vi "AlliGator Run XY Graph Python Function (API v1).vi"(6 "Mouse Click Event Data":T1, 7 "AlliGator Ctrl Refnums":T8, 8 "error in (no error)":errorcluster, 9 "data value reference in":refnum<data-value>, 10 "Python Function Info":T4, 11 "Python Session ID":refnum<k35>) -> (0 "error out":errorcluster, 1 "Data Value Reference out":refnum<data-value>, 2 "JSON String":string, 3 "Function Display Name":string, 4 "Function Parameters JSON String":string, 5 "Message":string)   [LabVIEW 2021, in "AlliGator Python Plugins.lvlib"]
uses:
  AlliGator Python Plugins.lvlib
  GUI/AlliGator Ctrl Refnums.ctl
  GUI/AlliGator Other Ctrl Refnums.ctl
  GUI/AlliGator State Indicator.ctl
  GUI/AlliGator Main Window Tabs.ctl
  GUI/AlliGator Phasor Plot Ctrl Refnums.ctl
  GUI/AlliGator Phasor Graph Ctrl Refnums.ctl
  Phasor/Phasor Calibration Type.ctl
  GUI/AlliGator Dataset Ctrl Refnums.ctl
  Source Image/AlliGator Displayed Image.ctl
  GUI/AlliGator Registered Events Ctrl Refnums.ctl
  GUI/AlliGator Image Histogram Control Refnums.ctl
  Histograms/Linear Histogram Options.ctl
  Histograms/Histogram Bin Option.ctl
  Histograms/Histogram Bin Position.ctl
  Decay Fit Parameter Map/AlliGator Decay Fit Map Control Refnums.ctl
  Fits/IRF(X)PSED/Decay Fit Parameters & Derived Quantities List v2.ctl
  Parameter Map/AlliGator Parameter Map Control Refnums.ctl
  Internal Variables/AlliGator Internal Variables v2.ctl
  <vilib>/vision/Image Controls.llb/IMAQ Image.ctl
  Internal Variables/AlliGator Gate Image Set.ctl
  Files/AlliGator FLI Dataset Type.ctl
  Files/AlliGator Data Series Type.ctl
  Dual-Channel Datasets/AlliGator Dataset Channel.ctl
  Settings/AlliGator Gate Arithmetic.ctl
  Image/Named ROI Description.ctl
  Phasor Graph/AlliGator Decay Metadata v3.ctl
  Decay Analysis/Decay Preprocessing/AlliGator Decay Background Subtraction Info.ctl
  Decay Analysis/Decay Preprocessing/AlliGator Baseline Subtraction Method.ctl
  Graphs/XY Graph/XY Graph Plot Shift Parameters.ctl
  Graphs/XY Graph/XY Graph Plot Shift Method.ctl
  Decay Analysis/Decay Preprocessing/AlliGator Decay Extrapolation Parameters.ctl
  Phasor/Calibration Phasor (m, phi).ctl
  Phasor/Phasor Reference Series.ctl
  Phasor/Phasor Calibration Map v2.ctl
  Phasor/Phasor (g, s).ctl
  Phasor Graph/AlliGator Raw Phasor Plot Data v5.ctl
  Phasor/Phasor Standard Deviation Options.ctl
  Phasor Plot/AlliGator Phasor Multi-Harmonic Data.ctl
  Phasor/Phasor Harmonic Data.ctl
  Decay Fit Parameter Map/AlliGator Decay Fit Options & Parameters v4.ctl
  Fits/IRF(X)PSED/Decay Fit Options v4.ctl
  Fits/Decay Convolution/Decay Model.ctl
  Fits/Residual Type.ctl
  Fits/IRF(X)PSED/Fit Weights Type v2.ctl
  Fits/Non-linear Fitting Method v2.ctl
  Fits/Fit Calculation Method.ctl
  Fits/Non-linear Fitting Algorithm.ctl
  Decay Analysis/Decay Fit/AlliGator Decay Fit Parameter Constraints 2.ctl
  Fits/IRF(X)PSED/Decay Fit Parameters In List.ctl
  Fits/IRF(X)PSED/MLE Baseline Offset Type.ctl
  Decay Analysis/Decay Preprocessing/AlliGator Decay Preprocessing Parameters.ctl
  Fits/IRF(X)PSED/Decay Fit Result Constraint.ctl
  Decay Fit Parameter Map/AlliGator Parameter Maps Data.ctl
  AlliGator Python Function Information.ctl
  AlliGator Python Function Parameter Definition.ctl
  AlliGator Python Function Output Definition.ctl
  AlliGator Python Plugin Target Type.ctl
  Graphs/XY Graph/XY Graph Mouse Click Event Data.ctl
  Graphs/XY Graph/XY Graph Refnum.ctl
  <vilib>/Utility/miscctls.llb/LVPoint32TypeDef.ctl
  AlliGator Python Plugin Plot Data v1.ctl
  AlliGator Python Plugin Graph Data v1.ctl
  Graphs/Get Plot at Mouse Click (XY Graph)/Get Plot at Mouse Click [AAC].vi
  Graphs/Graphs.lvlib
  Graphs/XY Graph/XY Graph Add-Ons.lvlib
  Strings/Strings.lvlib
  GUI/AlliGator GUI.lvlib
  Error/Error.lvlib
  Source Image/AlliGator Source Image.lvlib
  Phasor/Phasor.lvlib
  Histograms/Histogram Window.lvlib
  Fits/Fits.lvlib
  Decay Fit Parameter Map/AlliGator Decay Fit Parameter Map.lvlib
  Parameter Map/AlliGator Parameter Map.lvlib
  Image/Image.lvlib
  Decay Analysis/Decay Preprocessing/AlliGator Decay Preprocessing.lvlib
  Phasor Graph/AlliGator Phasor Graph.lvlib
  Files/AlliGator Files.lvlib
  Internal Variables/AlliGator Internal Variables.lvlib
  Phasor Plot/AlliGator Phasor Plot.lvlib
  Decay Analysis/Decay Fit/AlliGator Decay Fit.lvlib
  Settings/AlliGator Settings.lvlib
  Dual-Channel Datasets/AlliGator Dual-Channel Datasets.lvlib
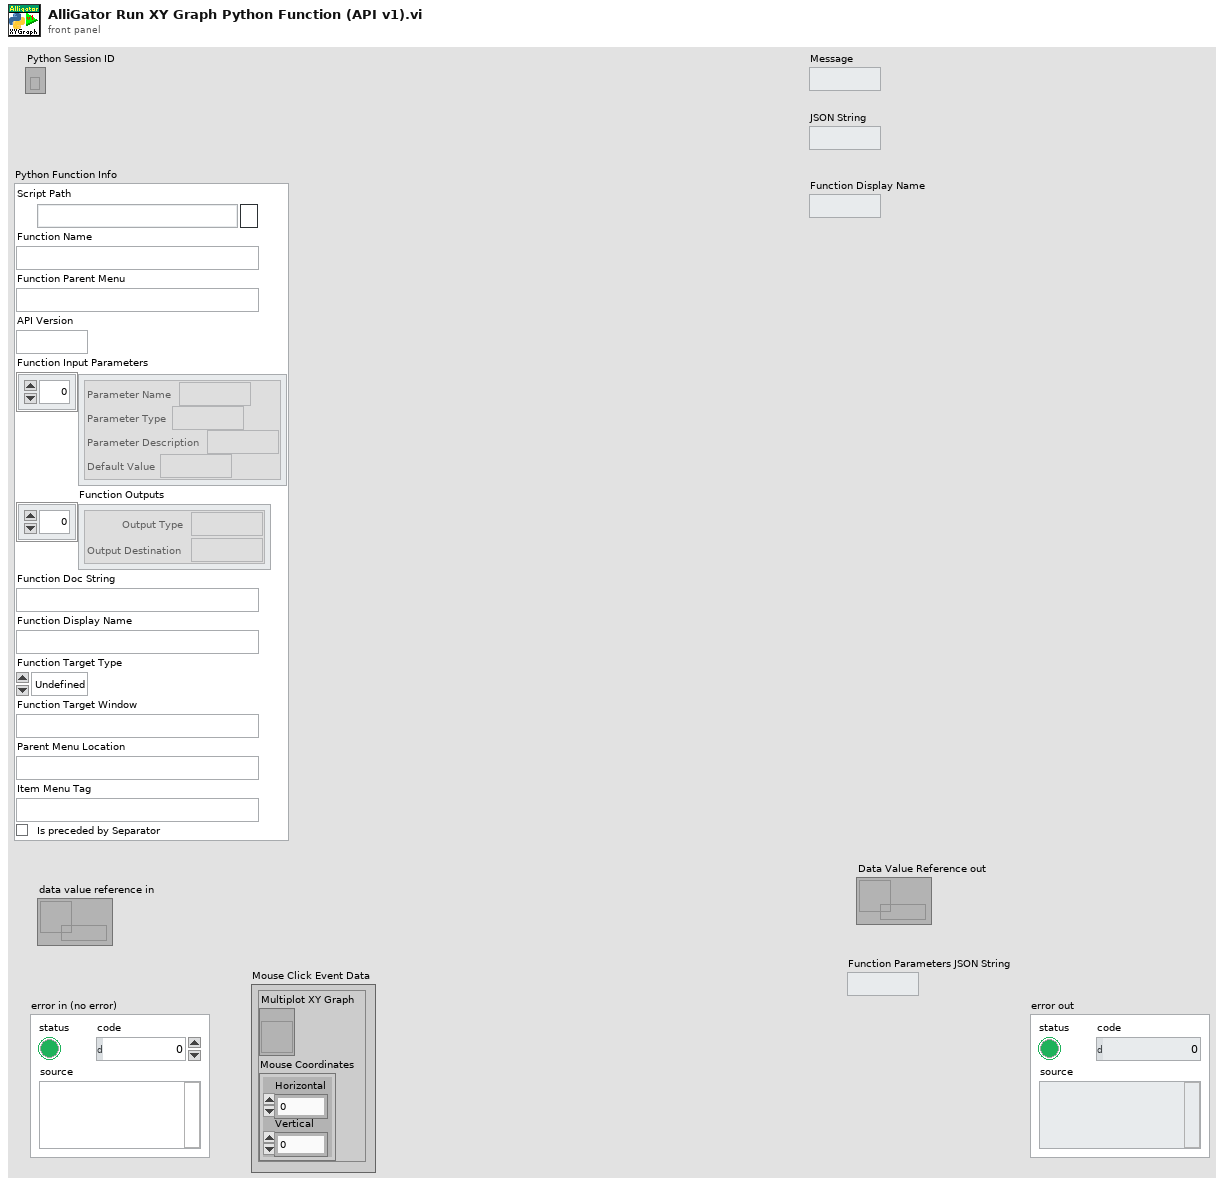
[diagram p1: front panel]
types:
  T1 = typedef "XY Graph Add-Ons.lvlib/XY Graph Mouse Click Event Data.ctl" = cluster{"Multiplot XY Graph":T2, "Mouse Coordinates":T3}
  T2 = typedef "XY Graph Add-Ons.lvlib/XY Graph Refnum.ctl" = refnum<vi>
  T3 = typedef "LVPoint32TypeDef.ctl" = cluster{"Horizontal":i32, "Vertical":i32}
  T4 = typedef "AlliGator Python Plugins.lvlib/AlliGator Python Function Information.ctl" = cluster{"Script Path":path, "Function Name":string, "Function Parent Menu":string, "API Version":string, "Function Input Parameters":T5[], "Function Outputs":T6[], "Function Doc String":string, "Function Display Name":string, "Function Target Type":T7, "Function Target Window":string, "Parent Menu Location":string, "Item Menu Tag":string, "Is preceded by Separator":bool}
  T5 = typedef "AlliGator Python Plugins.lvlib/AlliGator Python Function Parameter Definition.ctl" = cluster{"Parameter Name":string, "Parameter Type":string, "Parameter Description":string, "Default Value":string}
  T6 = typedef "AlliGator Python Plugins.lvlib/AlliGator Python Function Output Definition.ctl" = cluster{"Output Type":string, "Output Destination":string}
  T7 = typedef "AlliGator Python Plugins.lvlib/AlliGator Python Plugin Target Type.ctl" = enum16{"Undefined", "Window Menu", "Object Menu"}
  T8 = typedef "AlliGator GUI.lvlib/AlliGator Ctrl Refnums.ctl" = cluster{"Other AlliGator Ctrl Refnums":T9, "Phasor Plot Ctrl Refnums":T10, "Phasor Graph Ctrl Refnums":T11, "Dataset Control Refnums":T12, "Registered Events Ctrl Refnums":T13, "Image Histogram Ctrl Refnums":T14, "Decay Fit Map Ctrl Refnums":T15, "Parameter Map Ctrl Refnums":T16}
  T9 = typedef "AlliGator GUI.lvlib/AlliGator Other Ctrl Refnums.ctl" = cluster{"State Indicators":refnum<vi>, " Progress Bar":refnum<vi>, "Decay Graph Active":refnum<vi>, "Decay Statistics Bin":refnum<vi>, "Time Step":refnum<vi>, "Use File Timestamp":refnum<vi>, "Tab Control":refnum<vi>, "CPU":refnum<vi>, "Abort Fit":refnum<vi>, "Dataset File/Folder Path":refnum<vi>, "Abort ROI Creation":refnum<vi>, "Event LED":refnum<vi>, "Dataset File/Folder Path 2":refnum<vi>, "Dataset File/Folder Path 3":refnum<vi>, "Dataset File/Folder Path 4":refnum<vi>, "Dataset File/Folder Path 5":refnum<vi>, "Dataset File/Folder Path 6":refnum<vi>, "Dataset File/Folder Path 7":refnum<vi>, "Dataset File/Folder Path 8":refnum<vi>, "Dataset File/Folder Path 9":refnum<vi>, "Dataset File/Folder Path 10":refnum<vi>, "Dataset File/Folder Path 11":refnum<vi>}
  T10 = typedef "AlliGator GUI.lvlib/AlliGator Phasor Plot Ctrl Refnums.ctl" = cluster{"Phasor Ratio":refnum<vi>, "Modulus Lifetime":refnum<vi>, "Phasor at cursor (m, phi)":refnum<vi>, "Phase Lifetime":refnum<vi>, "Phasor at cursor (g, s)":refnum<vi>, "Phasor Plor Average Lifetime":refnum<vi>, "Phasor Plot Active":refnum<vi>, "Save Phasor Plot":refnum<vi>, "Image Overlay Color":refnum<vi>, "Phasor Plot Color Scale":refnum<vi>, "Reference 1 Button":refnum<vi>, "Reference 2 Button":refnum<vi>, "True Phasor Plot Value":refnum<vi>}
  T11 = typedef "AlliGator GUI.lvlib/AlliGator Phasor Graph Ctrl Refnums.ctl" = cluster{"Phasor Ratio":refnum<vi>, "Modulus Lifetime":refnum<vi>, "Phasor at cursor (m, phi)":refnum<vi>, "Phase Lifetime":refnum<vi>, "Phasor at cursor (g, s)":refnum<vi>, "Phasor Graph Average Lifetime":refnum<vi>, "Phasor Graph Active":refnum<vi>, "Save Phasor Graph":refnum<vi>, "Phasor Frame Slide":refnum<vi>, "Single Step Phasor":refnum<vi>, "Calibration Type":refnum<vi>, "Show Line":refnum<vi>, "Phase Lifetime 1":refnum<vi>, "Phase Lifetime 2":refnum<vi>, "Phasor Graph Frequency":refnum<vi>, "Phasor Reference 1 Control":refnum<vi>, "Phasor Reference 2 Control":refnum<vi>, "Calibration Lifetime":refnum<vi>, "Phase Lifetime SDV":refnum<vi>, "Average Lifetime SDV":refnum<vi>, "Phasor Ratio SDV":refnum<vi>, "Modulus Lifetime SDV":refnum<vi>}
  T12 = typedef "AlliGator GUI.lvlib/AlliGator Dataset Ctrl Refnums.ctl" = cluster{"Current Data":refnum<vi>, "Gate Image Slide":refnum<vi>, "Time Point Slide":refnum<vi>, "Current Time Stamp":refnum<vi>, "Save Image":refnum<vi>, "Displayed Image":refnum<vi>, "Overlay Mode":refnum<vi>, "Phasor Overlay Color":refnum<vi>, "Image Color Scale":refnum<vi>, "Use ROI as Search Area":refnum<vi>, "Source Image ROI Color":refnum<vi>, "True Pixel Value":refnum<vi>}
  T13 = typedef "AlliGator GUI.lvlib/AlliGator Registered Events Ctrl Refnums.ctl" = cluster{"Time Point Slider":refnum<vi>, "Phasor Plot Display Range":refnum<vi>, "Decay Graph":refnum<vi>, "Decay Statistics Graph":refnum<vi>, "Intensity Time Trace":refnum<vi>, "Phasor Graph":refnum<vi>, "Phasor Ratio Graph":refnum<vi>, "Lifetime Graph":refnum<vi>, "Phasor Plot Display":refnum<vi>, "Source Image Display":refnum<vi>, "Decay Fit Parameter Map Display Range":refnum<vi>, "Decay Fit Parameter Map Display":refnum<vi>, "Parameter Map Display Range":refnum<vi>, "Parameter Map Display":refnum<vi>, "Phasor Plot Display Range":refnum<vi>}
  T14 = typedef "AlliGator GUI.lvlib/AlliGator Image Histogram Control Refnums.ctl" = cluster{"Image Histogram":refnum<vi>, "Image Histogram Options":refnum<vi>, "Image Histogram Active":refnum<vi>, "Image Histogram Upper Percentile":refnum<vi>, "Image Histogram Lower Percentile":refnum<vi>, "Auto-Adjust Contrast":refnum<vi>}
  T15 = typedef "AlliGator Decay Fit Parameter Map.lvlib/AlliGator Decay Fit Map Control Refnums.ctl" = cluster{"Decay Fit Parameter Map Color Scale":refnum<vi>, "Decay Fit Parameter":refnum<vi>, "Max Parameter":refnum<vi>, "Min Parameter":refnum<vi>, "Decay Fit Parameter Map Display":refnum<vi>, "Decay Fit Parameter Map Display Range":refnum<vi>, "Decay Parameter Map X":refnum<vi>, "Decay Parameter Map Y":refnum<vi>, "Decay Parameter Map Value":refnum<vi>}
  T16 = typedef "AlliGator Parameter Map.lvlib/AlliGator Parameter Map Control Refnums.ctl" = cluster{"Parameter Map Color Scale":refnum<vi>, "Map Parameter":refnum<vi>, "Max Parameter":refnum<vi>, "Min Parameter":refnum<vi>, "Parameter Map Display":refnum<vi>, "Parameter Map Display Range":refnum<vi>, "Parameter Map Set":refnum<vi>, "Parameter Map X":refnum<vi>, "Parameter Map Y":refnum<vi>, "Parameter Map Value":refnum<vi>}
  T17 = typedef "AlliGator Python Plugins.lvlib/AlliGator Python Plugin Graph Data v1.ctl" = cluster{"Graph_Name":string, "Plots":T18[], "Reference_Decay":T18}
  T18 = typedef "AlliGator Python Plugins.lvlib/AlliGator Python Plugin Plot Data v1.ctl" = cluster{"Plot_Name":string, "X_Array":dbl[], "Y_Array":dbl[]}
  T19 = typedef "AlliGator Python Plugins.lvlib/AlliGator Type of Plot Data.ctl" = enum16{"Single Plot", "Selected Plots", "All Plots"}
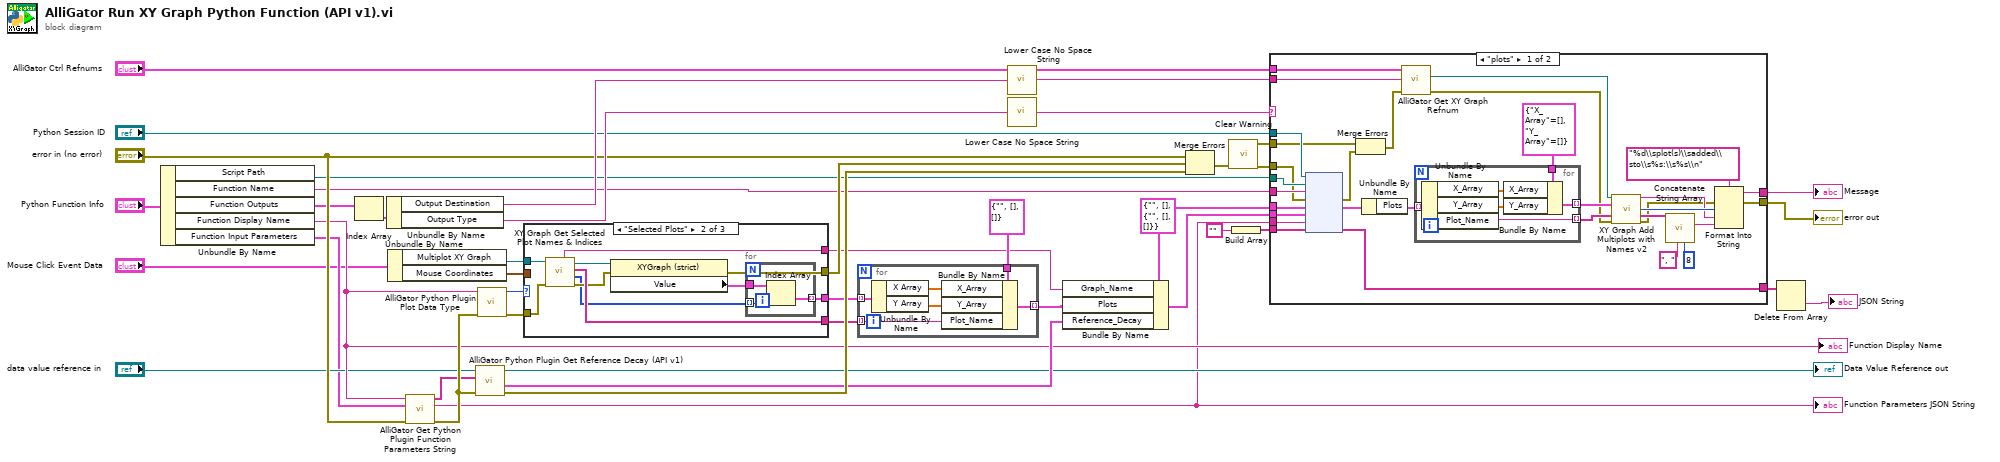
[diagram p0: block diagram]
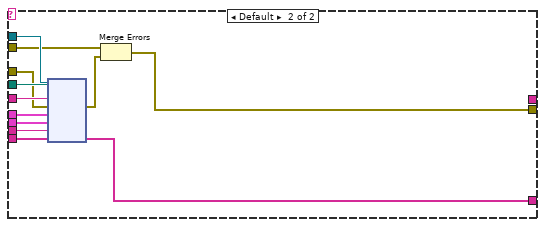
[diagram p2: hidden frame]
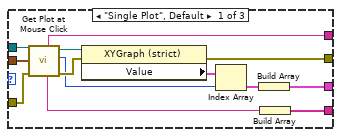
[diagram p3: hidden frame]
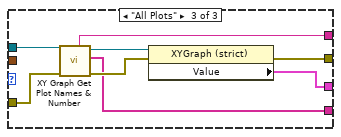
[diagram p4: hidden frame]
diagram:
  w29 = T17 {"Graph_Name"="", "Plots"=[], "Reference_Decay"={"Plot_Name"="", "X_Array"=[], "Y_Array"=[]}} ("Graph Plugin Data")
  n1 = Unbundle By Name("Python Function Info") -> ("Script Path"=w5:path, "Function Name"=w8:string, "Function Outputs"=w11:T6[], "Function Display Name"=w10:string, "Function Input Parameters"=w6:T5[])
  "Function Display Name" <- w10
  n2 = Index Array(array=w11) -> (element=w37:T6)  [unwired: 1 in]
  n3 = Unbundle By Name(w37) -> ("Output Destination"=w40:string, "Output Type"=w38:string)
  n4 = Unbundle By Name("Mouse Click Event Data") -> ("Multiplot XY Graph"=w17:T2, "Mouse Coordinates"=w18:T3)
  n5 = call "AlliGator Get Python Plugin Function Parameters String.vi"("error in (no error)"="error in (no error)", "Function Parameters"=w6, "Function Display Name"=w10) -> ("error out"=w26:errorcluster, "Function Parameters JSON String"=w3:string, "Parameter Names Not Found"=w25:string[])  [unwired: 6 in]
  "Function Parameters JSON String" <- w3
  n6 = call "AlliGator Python Plugin Get Reference Decay (API v1).vi"("error in (no error)"=w26, "AlliGator Parameter Names in"=w25, "Data Value Reference in"="data value reference in") -> ("error out"=w43:errorcluster, "Reference Decay"=w27:T18, "Data Value Reference out"=→"Data Value Reference out":refnum<data-value>)  [unwired: 4 in, 2 out]
  n7 = call "AlliGator Python Plugin Plot Data Type.vi"("error in (no error)"=w26, "Function Name"=w10) -> ("error out"=w20:errorcluster, "Type of Plot Data"=w19:T19)  [unwired: 8 in]
  n8 = case shown="\"Selected Plots\"" w19 {
    tunnel: w17 -> [w52 w66 w75]
    tunnel: w18 -> [w51 _ _]
    tunnel: [w50 w57 w76] -> w42
    tunnel: [w47 w63 w70] -> w23
    tunnel: w20 -> [w48 w65 w74]
    tunnel: [w46 w58 w77] -> w22
    tunnel: [w45 w64 w71] -> w21
    frame "Single Plot", Default {
      n9 = call-poly "Get Plot at Mouse Click.vi"("error in (no error)"=w48, "Mouse Click Coordinates"=w51, "XY Graph in"=w52) -> ("error out"=w55:errorcluster, "Plot at Coordinates"=w53:i32, "XY Graph out"=w56:T2, "Plot Name"=w49:string, "Graph Name"=w45:string)  [unwired: 2 in, 2 out]
      n10 = property class="XYGraph (strict)"(reference=w56, error in=w55) -> (error out=w50:errorcluster, "Value"=w54:cluster{"X Array":dbl[], "Y Array":dbl[]}[])  [unwired: 1 out]
      n11 = Index Array(array=w54, index=w53) -> (element=w44:cluster{"X Array":dbl[], "Y Array":dbl[]})
      n12 = Build Array(w44) -> (w46:cluster{"X Array":dbl[], "Y Array":dbl[]}[])
      n13 = Build Array(w49) -> (w47:string[])
    }
    frame "Selected Plots" {
      n14 = call "XY Graph Get Selected Plot Names & Indices.vi"("error in (no error)"=w65, "XY Graph in"=w66) -> ("error out"=w62:errorcluster, "Selected Plot Indices"=w60:i32[], "Selected Plot Names"=w63:string[], "XY Graph out"=w61:T2, "Graph Name"=w64:string)  [unwired: 5 in]
      n15 = property class="XYGraph (strict)"(reference=w61, error in=w62) -> (error out=w57:errorcluster, "Value"=w59:cluster{"X Array":dbl[], "Y Array":dbl[]}[])  [unwired: 1 out]
      n16 = for {
        tunnel: w60 -> [w69] mode=indexing
        tunnel: w59 -> [w68]
        tunnel: [w67] -> w58 mode=indexing
        n17 = Index Array(array=w68, index=w69) -> (element=w67:cluster{"X Array":dbl[], "Y Array":dbl[]})
      }
    }
    frame "All Plots" {
      n18 = call "XY Graph Get Plot Names & Number.vi"("error in (no error)"=w74, "XYGraph in"=w75) -> ("error out"=w73:errorcluster, "Plot Names"=w70:string[], "XYGraph out"=w72:T2, "Graph Name"=w71:string)  [unwired: 4 in, 2 out]
      n19 = property class="XYGraph (strict)"(reference=w72, error in=w73) -> (error out=w76:errorcluster, "Value"=w77:cluster{"X Array":dbl[], "Y Array":dbl[]}[])  [unwired: 1 out]
    }
  }
  n20 = for {
    tunnel: w23 -> [w83] mode=indexing
    tunnel: [w82] -> w30 mode=indexing
    tunnel: w22 -> [w81] mode=indexing
    tunnel: T18 {"Plot_Name"="", "X_Array"=[], "Y_Array"=[]} ("Plugin Plot Data") -> [w78]
    n21 = Unbundle By Name(w81) -> ("X Array"=w80:dbl[], "Y Array"=w79:dbl[])
    n22 = Bundle By Name(cluster=w78, "X_Array"=w80, "Y_Array"=w79, "Plot_Name"=w83) -> (w82:T18)
  }
  n23 = call "Lower Case No Space String.vi"("String"=w40) -> ("Lower Case No Space String"=w41:string)
  n24 = call "Lower Case No Space String.vi"("String"=w38) -> ("Lower Case No Space String"=w39:string)
  n25 = Bundle By Name(cluster=w29, "Graph_Name"=w21, "Plots"=w30, "Reference_Decay"=w27) -> (w28:T17)
  n26 = Merge Errors("error in (no error)", w42, w43) -> (w34:errorcluster)
  n27 = call "Clear Warning.vi"("error in (no error)"=w34) -> ("cleared warning or error dup"=w35:errorcluster, "error in (dup)"=w36:errorcluster)  [unwired: 9 in]
  n28 = Build Array("") -> (w33:string[])
  n29 = case shown="\"plots\"" w39 {
    tunnel: "Python Session ID" -> [w114 w132]
    tunnel: w3 -> [w113 w131]
    tunnel: w5 -> [w109 w130]
    tunnel: [w108 w129] -> w24
    tunnel: w8 -> [w106 w127]
    tunnel: w28 -> [w102 w126]
    tunnel: w29 -> [w101 w125]
    tunnel: w33 -> [w98 w124]
    tunnel: w35 -> [w97 w123]
    tunnel: w36 -> [w96 w122]
    tunnel: [w90 _] -> w12
    tunnel: [w89 w121] -> w13
    tunnel: w41 -> [w86 _]
    tunnel: "AlliGator Ctrl Refnums" -> [w84 _]
    frame "plots" {
      n30 = node(w114, w109, w106, w97, w101, w102, w113, w98) -> (w107:errorcluster, w112:T17, w108:string[])  [unwired: 2 in, 3 out]
      n31 = Merge Errors(w96, w107) -> (w88:errorcluster)
      n32 = Unbundle By Name(w112) -> ("Plots"=w99:T18[])
      n33 = call "AlliGator Get XY Graph Refnum.vi"("error in (no error)"=w88, "XY Graph Name"=w86, "AlliGator Ctrl Refnums"=w84) -> ("error out"=w87:errorcluster, "XY Graph reference"=w85:T2)  [unwired: 7 in]
      n34 = for {
        tunnel: w99 -> [w120] mode=indexing
        tunnel: [w119] -> w110 mode=indexing
        tunnel: cluster{"X_Array":dbl[], "Y_Array":dbl[]} {"X_Array"=[], "Y_Array"=[]} -> [w117]
        tunnel: [w115] -> w111 mode=indexing
        n35 = Unbundle By Name(w120) -> ("X_Array"=w118:dbl[], "Y_Array"=w116:dbl[], "Plot_Name"=w119:string)
        n36 = Bundle By Name(cluster=w117, "X_Array"=w118, "Y_Array"=w116) -> (w115:cluster{"X_Array":dbl[], "Y_Array":dbl[]})
      }
      n37 = call "XY Graph Add Multiplots with Names v2.vi"("XYGraph in"=w85, "Array of Plots"=w111, "Array of Plot Names (\"Plot\")"=w110, "error in (no error)"=w87) -> ("XY Graph Caption (or Label)"=w93:string, "Number of Plots Added"=w94:i32, "Added Plot Names"=w105:string[], "error out"=w91:errorcluster)  [unwired: 7 in, 1 out]
      n38 = call "Concatenate String Array.vi"("Max Number of Elements (None: -1)"=8, "Separator (TAB)"=", ", "String Array"=w105) -> ("Formatted String"=w92:string)  [unwired: 8 in]
      n39 = Format Into String(format string="%d\\splot(s)\\sadded\\sto\\s%s:\\s%s\\n", error in=w91, w94, w93, w92) -> (resulting string=w90:string, error out=w89:errorcluster)  [unwired: 1 in]
    }
    frame Default {
      n40 = node(w132, w130, w127, w123, w125, w126, w131, w124) -> (w128:errorcluster, w129:string[])  [unwired: 3 in, 3 out]
      n41 = Merge Errors(w122, w128) -> (w121:errorcluster)
    }
  }
  "error out" <- w13
  "Message" <- w12
  n42 = Delete From Array(array=w24) -> (deleted portion=→"JSON String":string)  [unwired: 2 in, 1 out]
